vi "Stop Test.vi"(8 "error in (no error)":errorcluster, 11 "XML Report In":refnum<class "XML Report.lvclass">) -> (0 "error out":errorcluster, 3 "XML Report Out":refnum<class "XML Report.lvclass">)   [LabVIEW 2020, in "XML Report.lvclass"]
uses:
  XML Report.lvclass
  Suite Result.ctl
  XML Report.lvclass/XML Report.ctl
  <vilib>/Utility/miscctls.llb/LVMapReplaceAction.ctl
  Core/Result/Status.ctl
  <vilib>/xml/Close Reference(Node).vi
  <vilib>/Platform/browser.llb/Open URL in Default Browser (path).vi
  <vilib>/xml/NI_XML.lvlib
  Core/Result/Result.lvlib
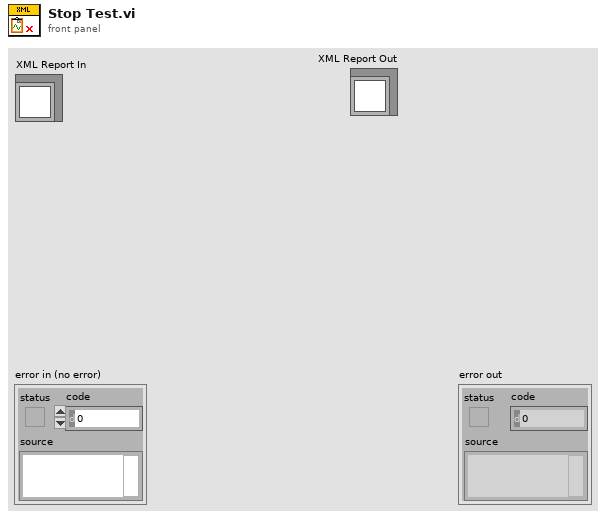
[diagram p1: front panel]
types:
  T1 = typedef "XML Report.lvclass/Suite Result.ctl" = cluster{"Name":string, "Tests":i32, "Failures":i32, "Execution Time":dbl}
  T2 = typedef "XML Report.lvclass/Case Result.ctl" = cluster{"Name":string, "Assertions":i32, "Classname":string, "Status":T3, "Time":dbl}
  T3 = typedef "Result.lvlib/Status.ctl" = enum16{"", "Passed", "Failed", "Error", "Skipped", "Setup Error", "Broken", "Teardown Error"}
  T4 = typedef "LVMapReplaceAction.ctl" = enum32{"Modify Entry only if found", "Add or Modify Entry", "Delete Entry"}
  T5 = typedef "Result.lvlib/Result.ctl" = cluster{"Name":string, "Description":string, "Status":T3, "Result Type":T6, "Execution Time":dbl, "Data":cluster{"Expected":variant, "Actual":variant, "Delta":variant}}
  T6 = typedef "Result.lvlib/Type.ctl" = enum16{"Test Case", "Test Suite", "Test Run", "Pass", "Fail", "Skip", "Pass if", "Fail if", "Pass if Error", "Fail if Error", "Pass if Equal", "Fail if Equal"}
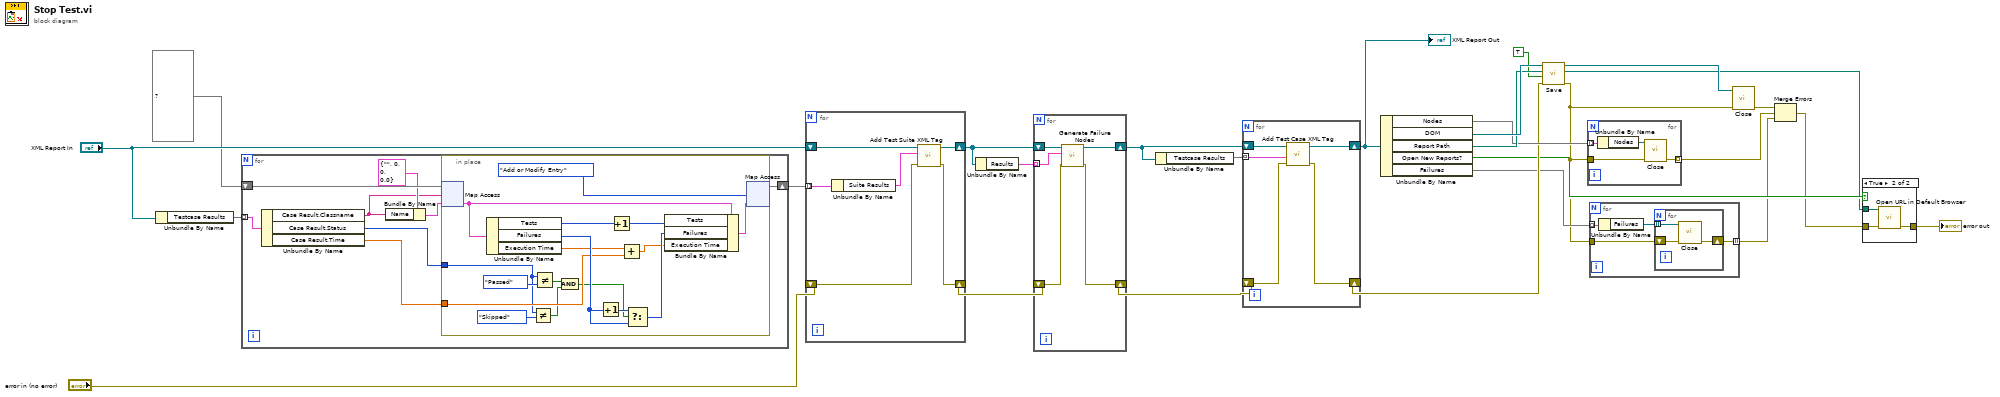
[diagram p0: block diagram]
diagram:
  n1 = Unbundle By Name("XML Report In") -> ("Testcase Results"=w14:map{string, T2})
  n2 = for {
    tunnel: w14 -> [w35] mode=indexing
    shift-right: [w34] -> w15
    shift-left: map{string, T1} {} ("map") -> [w33]
    n3 = Unbundle By Name(w35) -> ("Case Result.Classname"=w31:string, "Case Result.Status"=w29:T3, "Case Result.Time"=w28:dbl)
    n4 = Bundle By Name(cluster=T1 {"Name"="", "Tests"=0, "Failures"=0, "Execution Time"=0.0} ("value"), "Name"=w31) -> (w30:T1)
    n5 = in-place {
      in-place-border: w29 -> [w38]
      in-place-border: w28 -> [w42]
      n6 = in-place-map #1(w33, w31, w30) -> (w51:T1)  [unwired: 1 out]
      n7 = Unbundle By Name(w51) -> ("Tests"=w49:i32, "Failures"=w46:i32, "Execution Time"=w44:dbl)
      n8 = Not Equal?(x=w38, y=Status."Skipped" ("Status")) -> (x != y?=w37:bool)
      n9 = Not Equal?(x=w38, y=Status."Passed" ("Status")) -> (x != y?=w40:bool)
      n10 = And(x=w40, y=w37) -> (x .and. y?=w36:bool)
      n11 = Increment(x=w46) -> (x+1=w47:i32)
      n12 = Increment(x=w49) -> (x+1=w48:i32)
      n13 = Add(x=w44, y=w42) -> (x+y=w43:dbl)
      n14 = Select(t=w47, s=w36, f=w46) -> (s? t:f=w45:i32)
      n15 = Bundle By Name(cluster=w51, "Tests"=w48, "Failures"=w45, "Execution Time"=w43) -> (w50:T1)
      n16 = in-place-map #1(w50, LVMapReplaceAction."Add or Modify Entry" ("action")) -> (w34:map{string, T1})  [unwired: 2 out]
    }
  }
  n17 = for {
    shift-right: [w56] -> w5
    shift-left: "error in (no error)" -> [w57]
    shift-right: [w58] -> w7
    shift-left: "XML Report In" -> [w55]
    tunnel: w15 -> [w54] mode=indexing
    n18 = Unbundle By Name(w54) -> ("Suite Results"=w53:T1)
    n19 = call "Add Test Suite XML Tag.vi"("error in (no error)"=w57, "Suite Results"=w53, "Reports.lvlib:XML Report.lvclass"=w55) -> ("error out"=w56:errorcluster, "output cluster"=w58:refnum<class "XML Report.lvclass">)  [unwired: 7 in]
  }
  n20 = Unbundle By Name(w7) -> ("Results"=w6:T5[])
  n21 = for {
    shift-right: [w63] -> w8
    shift-left: w7 -> [w62]
    tunnel: w6 -> [w61] mode=indexing
    shift-right: [w59] -> w4
    shift-left: w5 -> [w60]
    n22 = call "Generate Failure Nodes.vi"("error in (no error)"=w60, "Result"=w61, "XML Report in"=w62) -> ("error out"=w59:errorcluster, "XML Report out"=w63:refnum<class "XML Report.lvclass">)  [unwired: 7 in]
  }
  n23 = Unbundle By Name(w8) -> ("Testcase Results"=w13:map{string, T2})
  n24 = for {
    shift-right: [w65] -> w20
    shift-left: w4 -> [w66]
    shift-right: [w67] -> w19
    shift-left: w8 -> [w68]
    tunnel: w13 -> [w64] mode=indexing
    n25 = call "Add Test Case XML Tag.vi"("error in (no error)"=w66, "Test Case Result"=w64, "Reports.lvlib:XML Report.lvclass"=w68) -> ("error out"=w65:errorcluster, "output cluster"=w67:refnum<class "XML Report.lvclass">)  [unwired: 7 in]
  }
  "XML Report Out" <- w19
  n26 = Unbundle By Name(w19) -> ("Nodes"=w23:map{string, refnum<k20>}, "DOM"=w27:refnum<k20>, "Report Path"=w24:path, "Open New Reports?"=w12:bool, "Failures"=w3:map{string, refnum<k20>[]})
  n27 = call <vilib>:"Save.vi"("error in (no error)"=w20, "overwrite file (True)"=TRUE, "XML file path"=w24, "DOM document in"=w27) -> ("error out"=w1:errorcluster, "XML file path out"=w9:path, "DOM document out"=w26:refnum<k20>)  [unwired: 5 in]
  n28 = for {
    tunnel: w23 -> [w72] mode=indexing
    tunnel: [w70] -> w22 mode=indexing
    tunnel: w1 -> [w69]
    n29 = Unbundle By Name(w72) -> ("Nodes"=w71:refnum<k20>)
    n30 = call-poly <vilib>:"Close.vi"("error in (no error)"=w69, "node"=w71) -> ("error out"=w70:errorcluster)  [unwired: 7 in]
  }
  n31 = for {
    tunnel: w3 -> [w76] mode=indexing
    tunnel: [w75] -> w2 mode=indexing
    tunnel: w1 -> [w74]
    n32 = Unbundle By Name(w76) -> ("Failures"=w73:refnum<k20>[])
    n33 = for {
      tunnel: w73 -> [w77] mode=indexing
      shift-right: [w79] -> w75
      shift-left: w74 -> [w78]
      n34 = call-poly <vilib>:"Close.vi"("error in (no error)"=w78, "node"=w77) -> ("error out"=w79:errorcluster)  [unwired: 7 in]
    }
  }
  n35 = call-poly <vilib>:"Close.vi"("error in (no error)"=w1, "node"=w26) -> ("error out"=w21:errorcluster)  [unwired: 7 in]
  n36 = Merge Errors(w21, w22, w2) -> (w11:errorcluster)
  n37 = case shown="True" w12 {
    tunnel: w9 -> [_ w81]
    tunnel: w11 -> [w80 w83]
    tunnel: [w80 w82] -> w10
    frame False {
    }
    frame True {
      n38 = call-poly <vilib>:"Open URL in Default Browser.vi"("error in (no error)"=w83, "path"=w81) -> ("error out"=w82:errorcluster)  [unwired: 4 in, 1 out]
    }
  }
  "error out" <- w10
